vi "Calc Text Rect_modded.vi"(4 "xy axis":T4={"x minimum"=0.0, "x maximum"=0.0, "x log?"=FALSE, "x precision"=1, "x format"=enum."Decimal", "y minimum"=0.0, "y maximum"=0.0, "y log?"=FALSE, "y precision"=1, "y format"=enum."Decimal"} {"x minimum" format="%.2f"; "x maximum" format="%.2f"; "y minimum" format="%.2f"; "y maximum" format="%.2f"}, 5 "desired font(Application)":T2(ring)=enum."Application Font", 6 "[user-specified font]":T3) -> (3 "y rect":T1, 7 "x rect":T1)   [LabVIEW 2018]
uses:
  fmt_prec_modded.ctl
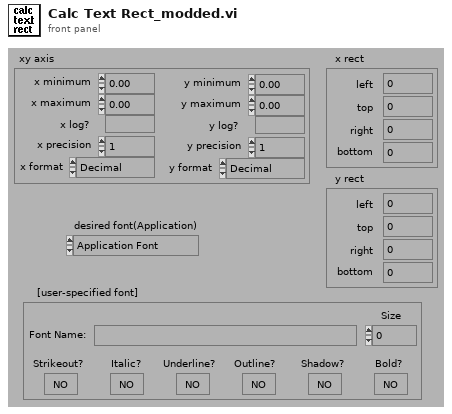
[diagram p1: front panel]
types:
  T1 = cluster{"left":i16, "top":i16, "right":i16, "bottom":i16}
  T2 = enum16{"User-specified Font", "Application Font", "System Font", "Dialog Font"}
  T3 = cluster{"Font Name:":string, "Size":i16, "Strikeout?":bool, "Italic?":bool, "Underline?":bool, "Outline?":bool, "Shadow?":bool, "Bold?":bool}
  T4 = cluster{"x minimum":dbl, "x maximum":dbl, "x log?":bool, "x precision":u8, "x format":enum8{"Decimal", "Scientific", "Engineering", "Binary", "Octal", "Hex", "Timestamp"}, "y minimum":dbl, "y maximum":dbl, "y log?":bool, "y precision":u8, "y format":enum8{"Decimal", "Scientific", "Engineering", "Binary", "Octal", "Hex", "Timestamp"}}
  T5 = typedef "fmt_prec_modded.ctl" = cluster{"format":enum8{"Decimal", "Scientific", "Engineering", "Binary", "Octal", "Hex", "Timestamp"}, "precision":u8}
  T6 = enum8{"Decimal", "Scientific", "Engineering", "Binary", "Octal", "Hex", "Timestamp"}
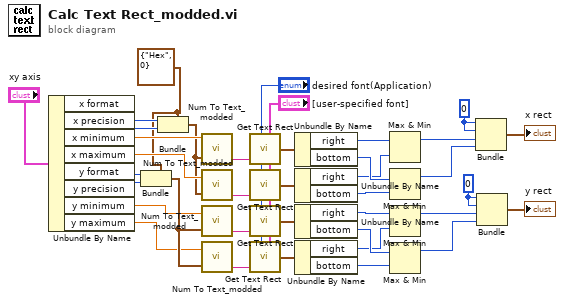
[diagram p0: block diagram]
diagram:
  w1 = T5 {"format"=enum."Hex", "precision"=0} ("fmt and prec")
  w14 = i16 0
  w17 = i16 0
  n1 = Unbundle By Name("xy axis") -> ("x format"=w5:T6, "x precision"=w6:u8, "x minimum"=w37:dbl, "x maximum"=w36:dbl, "y format"=w4:T6, "y precision"=w3:u8, "y minimum"=w35:dbl, "y maximum"=w34:dbl)
  n2 = Bundle(cluster=w1, "format"=w4, "precision"=w3) -> (w38:T5)
  n3 = Bundle(cluster=w1, "format"=w5, "precision"=w6) -> (w2:T5)
  n4 = call "Num To Text_modded.vi"("fmt and prec"=w2, "number"=w37) -> ("numeric string"=w33:string)
  n5 = call "Num To Text_modded.vi"("fmt and prec"=w2, "number"=w36) -> ("numeric string"=w32:string)
  n6 = call "Num To Text_modded.vi"("fmt and prec"=w38, "number"=w35) -> ("numeric string"=w31:string)
  n7 = call "Num To Text_modded.vi"("fmt and prec"=w38, "number"=w34) -> ("numeric string"=w30:string)
  n8 = call <vilib>:"Get Text Rect.vi"("desired font(Application)"="desired font(Application)", "text"=w33, "[user-specified font]"="[user-specified font]") -> ("rect"=w29:T1)  [unwired: 6 in]
  n9 = call <vilib>:"Get Text Rect.vi"("desired font(Application)"="desired font(Application)", "text"=w32, "[user-specified font]"="[user-specified font]") -> ("rect"=w28:T1)  [unwired: 6 in]
  n10 = call <vilib>:"Get Text Rect.vi"("desired font(Application)"="desired font(Application)", "text"=w31, "[user-specified font]"="[user-specified font]") -> ("rect"=w27:T1)  [unwired: 6 in]
  n11 = call <vilib>:"Get Text Rect.vi"("desired font(Application)"="desired font(Application)", "text"=w30, "[user-specified font]"="[user-specified font]") -> ("rect"=w26:T1)  [unwired: 6 in]
  n12 = Unbundle By Name(w29) -> ("right"=w25:i16, "bottom"=w23:i16)
  n13 = Unbundle By Name(w28) -> ("right"=w22:i16, "bottom"=w21:i16)
  n14 = Unbundle By Name(w27) -> ("right"=w24:i16, "bottom"=w19:i16)
  n15 = Unbundle By Name(w26) -> ("right"=w18:i16, "bottom"=w20:i16)
  n16 = Max & Min(x=w25, y=w22) -> (max(x,y)=w16:i16)  [unwired: 1 out]
  n17 = Max & Min(x=w23, y=w21) -> (max(x,y)=w15:i16)  [unwired: 1 out]
  n18 = Max & Min(x=w24, y=w18) -> (max(x,y)=w13:i16)  [unwired: 1 out]
  n19 = Max & Min(x=w19, y=w20) -> (max(x,y)=w12:i16)  [unwired: 1 out]
  n20 = Bundle(w17, w17, "right"=w16, "bottom"=w15) -> (→"x rect":cluster{i16, i16, "right":i16, "bottom":i16})  [unwired: 1 in]
  n21 = Bundle(w14, w14, "right"=w13, "bottom"=w12) -> (→"y rect":cluster{i16, i16, "right":i16, "bottom":i16})  [unwired: 1 in]
